vi "SubVI_for_assignment3.vi"(1 "Time interval":dbl, 2 "Frequency":dbl, 3 "Amplitude":dbl, 4 "Signal type":u32) -> (0 "Signal Output":dbl)   [LabVIEW 2017]
uses:
  <vilib>/ptbypt/NI_PtbyPt.lvlib
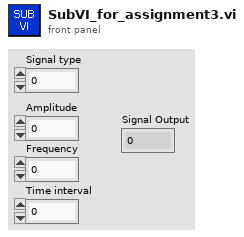
[diagram p1: front panel]
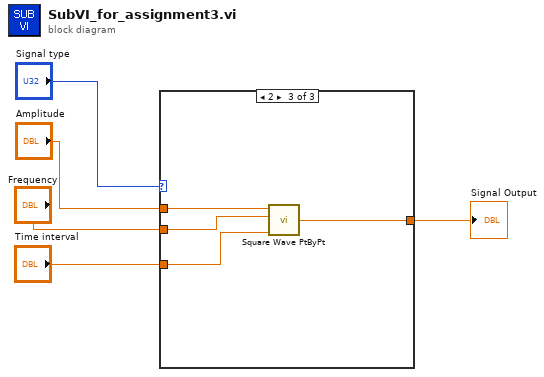
[diagram p0: block diagram]
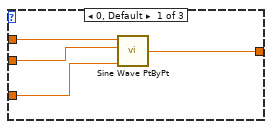
[diagram p2: hidden frame]
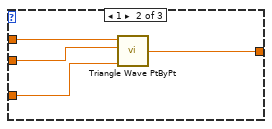
[diagram p3: hidden frame]
diagram:
  n1 = case shown="2" "Signal type" {
    tunnel: "Amplitude" -> [w9 w13 w17]
    tunnel: "Frequency" -> [w8 w12 w16]
    tunnel: "Time interval" -> [w7 w11 w15]
    tunnel: [w6 w10 w14] -> w1
    frame 0, Default {
      n2 = call <vilib>:"Sine Wave PtByPt.vi"("time"=w7, "frequency"=w8, "amplitude"=w9) -> ("sine wave"=w6:dbl)  [unwired: 1 in]
    }
    frame 1 {
      n3 = call <vilib>:"Triangle Wave PtByPt.vi"("time"=w11, "frequency"=w12, "amplitude"=w13) -> ("triangle wave"=w10:dbl)  [unwired: 1 in]
    }
    frame 2 {
      n4 = call <vilib>:"Square Wave PtByPt.vi"("amplitude"=w17, "frequency"=w16, "time"=w15) -> ("square wave"=w14:dbl)  [unwired: 2 in]
    }
  }
  "Signal Output" <- w1
